vi "Configure Mask Test Characteristics.vi"(0 "VISA resource name":refnum<visa-resource-name>, 1 "Waveforms (1000)":i32=1000, 2 "Enable Measuring (F: Disable)":bool, 3 "Enable Saving (F: Disable)":bool, 5 "Termination Condition (0: Forever)":i32(ring) items=["Forever", "Sigma", "Time", "Waveforms"], 7 "Sigma Level (6.0)":dbl=6.0, 9 "Time (1.0)":dbl=1.0, 11 "error in (no error)":errorcluster, 12 "Enable Mask Test (F: Disable)":bool, 13 "Enable Stopping (F: Disable)":bool) -> (4 "VISA resource name out":refnum<visa-resource-name>, 15 "error out":errorcluster)   [LabVIEW 2016, in "Agilent 2000 3000 X-Series.lvlib"]
doc: "Configure the basic settings of mask test."
uses:
  Agilent 2000 3000 X-Series.lvlib
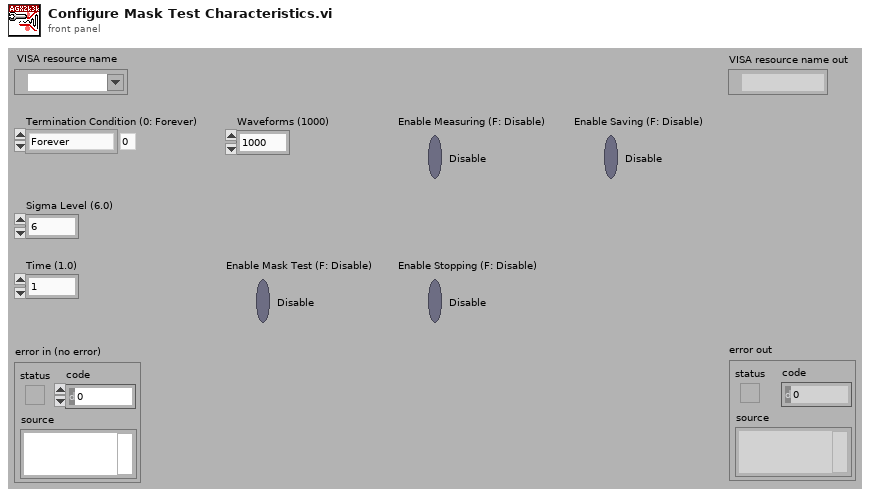
[diagram p1: front panel]
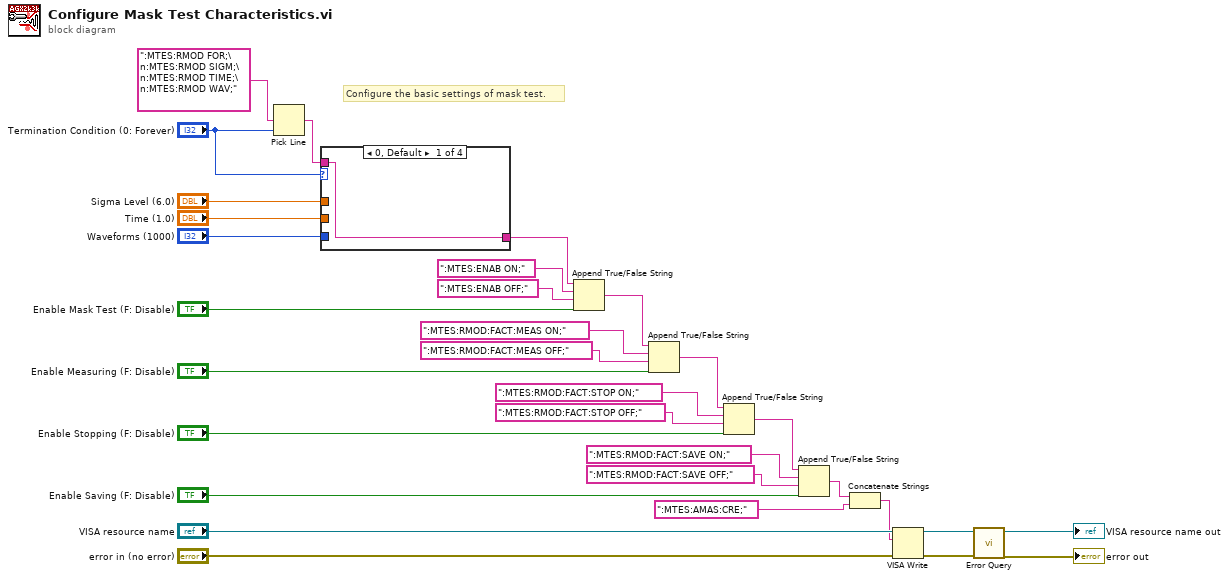
[diagram p0: block diagram]
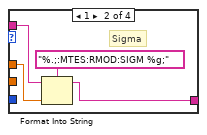
[diagram p2: hidden frame]
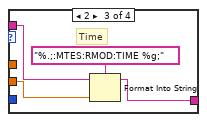
[diagram p3: hidden frame]
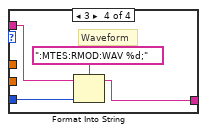
[diagram p4: hidden frame]
diagram:
  # "Configure the basic settings of mask test."
  n1 = Pick Line(multi-line string=":MTES:RMOD FOR;\n:MTES:RMOD SIGM;\n:MTES:RMOD TIME;\n:MTES:RMOD WAV;", line index="Termination Condition (0: Forever)") -> (output string=w2:string)  [unwired: 1 out]
  n2 = case shown="0, Default" "Termination Condition (0: Forever)" {
    tunnel: "Waveforms (1000)" -> [_ _ _ w43]
    tunnel: "Time (1.0)" -> [_ _ w40 _]
    tunnel: "Sigma Level (6.0)" -> [_ w36 _ _]
    tunnel: w2 -> [w32 w35 w39 w42]
    tunnel: [w32 w33 w37 w41] -> w1
    frame 0, Default {
    }
    frame 1 {
      # "Sigma"
      n3 = Format Into String(format string="%.;:MTES:RMOD:SIGM %g;", initial string=w35, w36) -> (resulting string=w33:string)  [unwired: 1 in, 1 out]
    }
    frame 2 {
      # "Time"
      n4 = Format Into String(format string="%.;:MTES:RMOD:TIME %g;", initial string=w39, w40) -> (resulting string=w37:string)  [unwired: 1 in, 1 out]
    }
    frame 3 {
      # "Waveform"
      n5 = Format Into String(format string=":MTES:RMOD:WAV %d;", initial string=w42, w43) -> (resulting string=w41:string)  [unwired: 1 in, 1 out]
    }
  }
  n6 = Append True/False String(1:"Enable Mask Test (F: Disable)", 2:":MTES:ENAB OFF;", 3:":MTES:ENAB ON;", 4:w1) -> (0:w27:string)
  n7 = Append True/False String(1:"Enable Measuring (F: Disable)", 2:":MTES:RMOD:FACT:MEAS OFF;", 3:":MTES:RMOD:FACT:MEAS ON;", 4:w27) -> (0:w23:string)
  n8 = Append True/False String(1:"Enable Stopping (F: Disable)", 2:":MTES:RMOD:FACT:STOP OFF;", 3:":MTES:RMOD:FACT:STOP ON;", 4:w23) -> (0:w19:string)
  n9 = Append True/False String(1:"Enable Saving (F: Disable)", 2:":MTES:RMOD:FACT:SAVE OFF;", 3:":MTES:RMOD:FACT:SAVE ON;", 4:w19) -> (0:w9:string)
  n10 = Concatenate Strings(w9, ":MTES:AMAS:CRE;") -> (w7:string)
  n11 = VISA Write(VISA resource name="VISA resource name", write buffer=w7, error in (no error)="error in (no error)") -> (VISA resource name out=w13:refnum<visa-resource-name>, error out=w12:errorcluster)  [unwired: 1 out]
  n12 = call "Error Query.vi"("error in (no error)"=w12, "VISA resource name"=w13) -> ("error out"=→"error out":errorcluster, "VISA resource name out"=→"VISA resource name out":refnum<visa-resource-name>)  [unwired: 8 out]
